vi "I2C Read.vi"(5 "EOF":T1, 6 "Timeout (1000 ms)":u16=1000, 7 "I2C Channel":u8, 8 "Error In":errorcluster, 9 "Bytes To Read":u8, 10 "I2C Slave Address (0)":u8, 11 "LINX Resource":T2) -> (0 "Error Out":errorcluster, 2 "Data":u8[](array[numeric]), 3 "LINX Resource":T2)   [LabVIEW 2011, in "LMH-LINX.lvlib"]
doc: "Read the specified number of bytes from the I2C slave on the specified channel."
uses:
  LMH-LINX.lvlib
  Private/Type Defs/LINX Ref.ctl
  Private/Type Defs/Platform.ctl
  Private/Type Defs/Interface.ctl
  Private/Device/Type Defs/LINX Device Config.ctl
  Private/Device/Type Defs/TCP Config.ctl
  Private/Device/Type Defs/Channels.ctl
  Private/Type Defs/Peripherals/I2C/EOF.ctl
  Private/Type Defs/Peripheral.ctl
  Private/Type Defs/Channel FGV States.ctl
  Private/Device/Device.lvlib
  <vilib>/myRIO/Instrument Drivers/Onboard IO/I2C/typedefs/I2C Reference.ctl
  <vilib>/myRIO/Instrument Drivers/Onboard IO/I2C/typedefs/I2C Configuration.ctl
  <vilib>/myRIO/Instrument Drivers/Onboard IO/I2C/typedefs/I2C Transfer Rate.ctl
  <vilib>/myRIO/Common/Instrument Driver Framework/myRIO v1.0/I2C/typedefs/I2C Channels Enum.ctl
  <vilib>/myRIO/Common/Instrument Driver Framework/Utilities/typedefs/myRIO Generic Hardware Reference.ctl
  <vilib>/myRIO/Common/Instrument Driver Framework/Utilities/typedefs/myRIO v1.0 Reference.ctl
  <vilib>/myRIO/Common/Instrument Driver Framework/Utilities/typedefs/Generic FPGA Reference.ctl
  <vilib>/myRIO/Common/Instrument Driver Framework/Utilities/typedefs/Hardware Version Enum.ctl
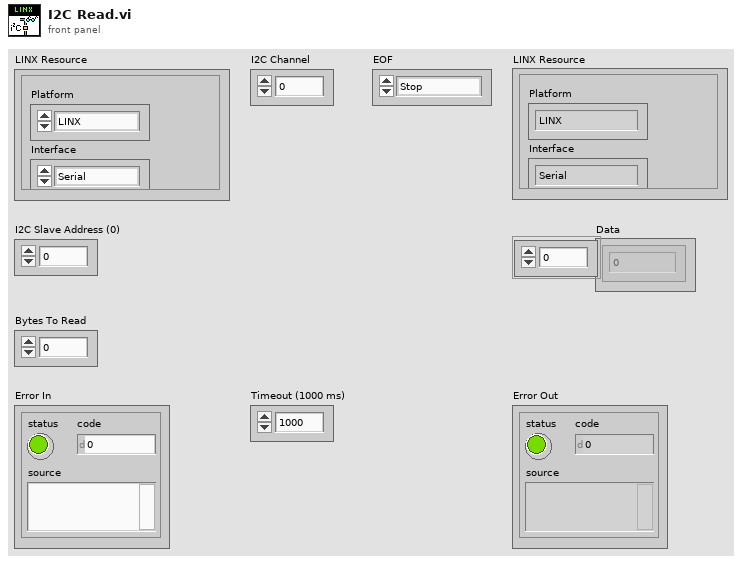
[diagram p1: front panel]
types:
  T1 = typedef "LMH-LINX.lvlib/EOF.ctl" = enum8{"Stop", "Restart", "Restart No Stop", "No Stop"}
  T2 = typedef "LMH-LINX.lvlib/LINX Ref.ctl" = cluster{"Platform":T3, "Interface":T4, "LINX Device Config":T5}
  T3 = typedef "LMH-LINX.lvlib/Platform.ctl" = enum16{"LINX", "myRIO"}
  T4 = typedef "LMH-LINX.lvlib/Interface.ctl" = enum16{"Serial", "TCP"}
  T5 = typedef "LMH-LINX.lvlib/Device.lvlib/LINX Device Config.ctl" = cluster{"Interface":T4, "COM Port":refnum<visa-resource-name>, "TCP Configuration":T6, "Device Family":u8, "Device ID":u8, "Device Name":string, "TCP Ref":refnum<k5>, "Channels":T7}
  T6 = typedef "LMH-LINX.lvlib/Device.lvlib/TCP Config.ctl" = cluster{"IP Address":string, "Port":u16}
  T7 = typedef "LMH-LINX.lvlib/Channels.ctl" = cluster{"DI":u8[], "DO":u8[], "AI":u8[], "AO":u8[], "PWM":u8[], "QE":u8[], "UART":u8[], "I2C 2":u8[], "SPI":u8[], "CAN":u8[], "Servo":u8[], "AI Ref (V)":dbl, "AO Ref (V)":dbl, "AO Resolution (Bits)":u8}
  T8 = typedef "LMH-LINX.lvlib/Peripheral.ctl" = enum8{"DI", "DO", "AI", "AO", "PWM", "QE", "UART", "I2C", "SPI", "CAN", "Servo"}
  T9 = typedef "LMH-LINX.lvlib/Channel FGV States.ctl" = enum16{"Initialize", "Get", "Set"}
  T10 = typedef "I2C.lvlib/I2C Reference.ctl" = cluster{"myRIO Reference":T11, "I2C Channels Enum":T15, "I2C Configuration":T16}
  T11 = typedef "myRIO Generic Hardware Reference.ctl" = cluster{"myRIO Model":T12, "myRIO Hardware Reference":T13}
  T12 = typedef "Hardware Version Enum.ctl" = enum16{"Unknown", "myRIO-1900", "myRIO-1950"}
  T13 = typedef "myRIO v1.0 Reference.ctl" = cluster{"Generic FPGA Reference":T14, "Allow multiple opens":bool}
  T14 = typedef "Generic FPGA Reference.ctl" = refnum<k20>
  T15 = typedef "I2C Channels Enum.ctl" = enum16{"Not Connected", "A/I2C", "B/I2C"}
  T16 = typedef "I2C.lvlib/I2C Configuration.ctl" = cluster{"I2C Transfer Rate":T17}
  T17 = typedef "I2C.lvlib/I2C Transfer Rate.ctl" = enum16{"Standard Mode (100 kbps)", "Fast Mode (400 kbps)"}
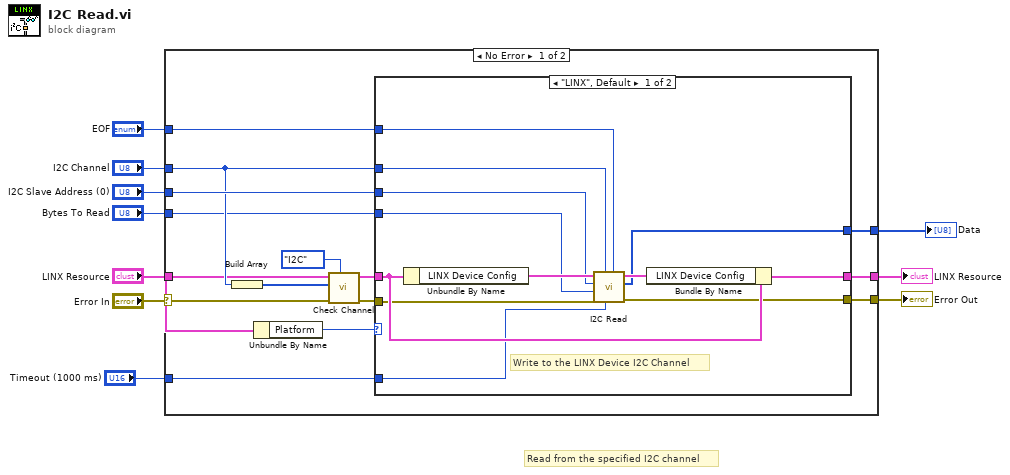
[diagram p0: block diagram]
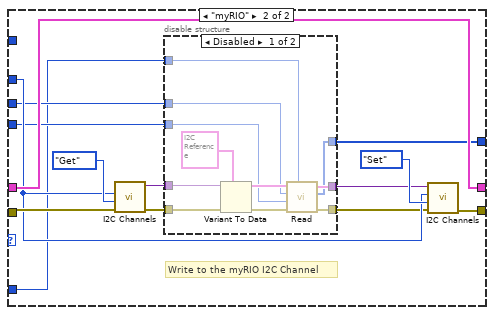
[diagram p2: hidden frame]
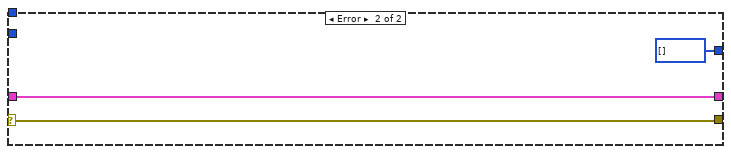
[diagram p4: hidden frame]
diagram:
  # "Read from the specified I2C channel"
  n1 = case shown="No Error" "Error In" {
    selector: "Error In" -> [w11 w65]
    tunnel: [w24 w65] -> w10
    tunnel: [w23 w64] -> w9
    tunnel: "I2C Slave Address (0)" -> [w22 _]
    tunnel: "I2C Channel" -> [w19 _]
    tunnel: "LINX Resource" -> [w17 w64]
    tunnel: "Bytes To Read" -> [w15 _]
    tunnel: [w14 u8[] [] ("Bytes Read")] -> w4
    tunnel: "Timeout (1000 ms)" -> [w13 _]
    tunnel: "EOF" -> [w12 _]
    frame No Error {
      n2 = Build Array(w19) -> (w18:u8[])
      n3 = Unbundle By Name(w17) -> ("Platform"=w25:T3)
      n4 = call "Check Channel.vi"("Peripheral"=Peripheral."I2C", "Error In"=w11, "Channels"=w18, "LINX Resource"=w17) -> ("Error Out"=w20:errorcluster, "LINX Resource"=w16:T2)  [unwired: 5 in, 1 out]
      n5 = case shown="\"LINX\", Default" w25 {
        tunnel: w20 -> [w33 w47]
        tunnel: w16 -> [w37 w51]
        tunnel: [w32 w50] -> w24
        tunnel: [w36 w51] -> w23
        tunnel: w19 -> [w31 w46]
        tunnel: w22 -> [w30 w43]
        tunnel: w15 -> [w29 w40]
        tunnel: [w28 w39] -> w14
        tunnel: w13 -> [w27 w38]
        tunnel: w12 -> [w26 _]
        frame "LINX", Default {
          # "Write to the LINX Device I2C Channel"
          n6 = Unbundle By Name(w37) -> ("LINX Device Config"=w35:T5)
          n7 = call "I2C Read.vi"("EOF"=w26, "Timeout (1000 ms)"=w27, "I2C Channel (0)"=w31, "Error In"=w33, "Bytes To Read"=w29, "I2C Slave Address"=w30, "LINX Device Config"=w35) -> ("Error Out"=w32:errorcluster, "Data"=w28:u8[], "LINX Device Config"=w34:T5)  [unwired: 2 in]
          n8 = Bundle By Name(cluster=w37, "LINX Device Config"=w34) -> (w36:T2)
        }
        frame "myRIO" {
          # "Write to the myRIO I2C Channel"
          n9 = call "I2C Channels.vi"("Error In"=w47, "Channel State"=Channel_FGV_States."Get", "Channel Number"=w46) -> ("Error Out"=w45:errorcluster, "I2C Channel"=w44:variant)  [unwired: 7 in]
          n10 = disable-structure shown="Disabled" {
            disable-tunnel: w45 -> [w61 _]
            disable-tunnel: w44 -> [w60 _]
            disable-tunnel: w43 -> [w54 _]
            disable-tunnel: [w58 _] -> w42
            disable-tunnel: [w57 _] -> w41
            disable-tunnel: w38 -> [w56 _]
            disable-tunnel: w40 -> [w53 _]
            disable-tunnel: [w52 _] -> w39
            frame Disabled {
              n11 = Variant To Data(error in=w61, type=T10 {"myRIO Reference"={"myRIO Model"=enum."Unknown", "myRIO Hardware Reference"={"Generic FPGA Reference"=refnum, "Allow multiple opens"=FALSE}}, "I2C Channels Enum"=enum."Not Connected", "I2C Configuration"={"I2C Transfer Rate"=enum."Standard Mode (100 kbps)"}}, Variant=w60) -> (data=w55:T10, error out=w59:errorcluster)
              n12 = call <vilib>:"Read.vi"("Timeout ms (1000)"=w56, "error in (no error)"=w59, "Byte Count"=w53, "Slave Address (7-bit)"=w54, "I2C Ref In"=w55) -> ("error out"=w57:errorcluster, "Bytes Read"=w52:u8[], "I2C Ref Out"=w58:T10)  [unwired: 3 in]
            }
            frame Enabled {
            }
          }
          n13 = call "I2C Channels.vi"("Error In"=w41, "Channel State"=Channel_FGV_States."Set", "Channel Number"=w46, "I2C Channel"=w42) -> ("Error Out"=w50:errorcluster)  [unwired: 6 in, 1 out]
        }
      }
    }
    frame Error {
    }
  }
  "Error Out" <- w10
  "LINX Resource" <- w9
  "Data" <- w4
